vi "Release Logs Queue.vi"(8 "Error In":errorcluster, 11 "EventLog in":refnum<class "LogsAbstract.lvclass">) -> (0 "Error Out":errorcluster, 3 "EventLog out":refnum<class "LogsAbstract.lvclass">)   [LabVIEW 2019, in "LogsAbstract.lvlib" / "LogsAbstract.lvclass"]
uses:
  LogsAbstract.lvclass
  Classes/Event/Event.lvclass
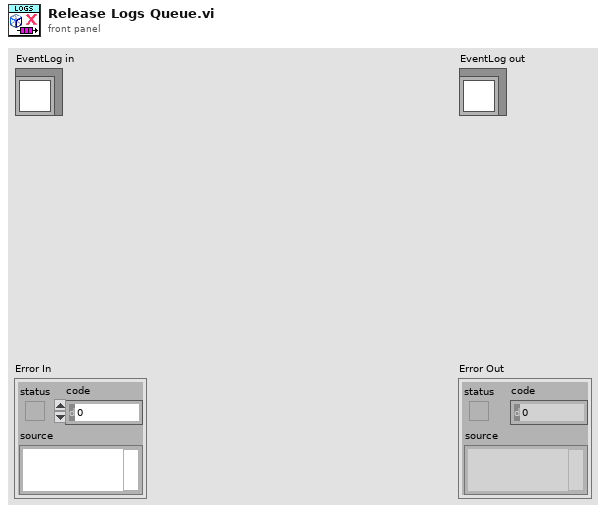
[diagram p1: front panel]
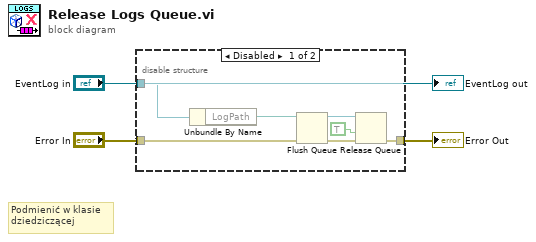
[diagram p0: block diagram]
diagram:
  # "Podmienić w klasie\ndziedziczącej"
  n1 = disable-structure shown="Disabled" {
    disable-tunnel: "Error In" -> [w10 w11]
    disable-tunnel: [w9 w11] -> w2
    disable-tunnel: "EventLog in" -> [w8 _]
    frame Disabled {
      n2 = Unbundle By Name(w8) -> ("LogPath"=w7:path)
      n3 = Flush Queue(queue=w7, error in (no error)=w10) -> (queue out=w6:refnum<queue>, error out=w5:errorcluster)  [unwired: 1 out]
      n4 = Release Queue(queue=w6, force destroy? (F)=TRUE, error in (no error)=w5) -> (error out=w9:errorcluster)  [unwired: 2 out]
    }
    frame Enabled {
    }
  }
  "Error Out" <- w2
  "EventLog out" <- "EventLog in"
